vi "Agilent Oscilloscope data download.vi"() -> ()   [LabVIEW 2011]
uses:
  <vilib>/Instr/_visa.llb/VISA Open Access Mode.ctl
  <vilib>/Instr/_visa.llb/VISA Set IO Buffer Mask.ctl
panel:
  in  "run time (ms)":u32=1000
  out "error out":errorcluster
  in  "VISA GPIB Resource":refnum<visa-resource-name>="GPIB0::7::INSTR"
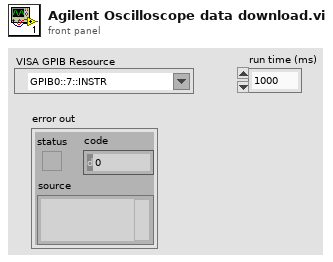
[diagram p1: front panel]
types:
  T1 = typedef "VISA Set IO Buffer Mask.ctl" = u16
  T2 = typedef "VISA Open Access Mode.ctl" = u32
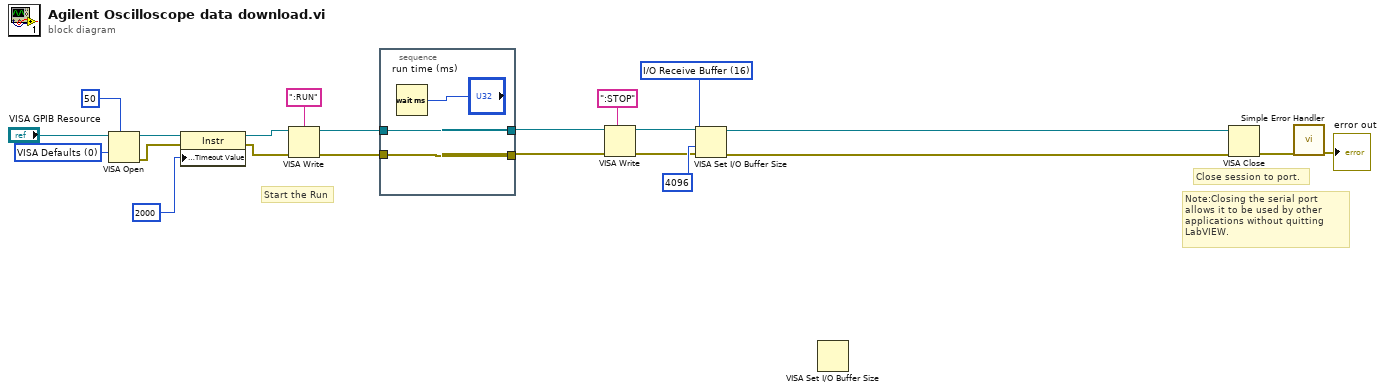
[diagram p0: block diagram]
diagram:
  w5 = T1 16 items=["I/O Receive Buffer"=16, "I/O Transmit Buffer"=32, "I/O Receive and Transmit Buffer"=48] ("Mask")
  w15 = T2 0 items=["VISA Defaults"=0, "Exclusive Lock"=1, "Load Configured Settings"=4] ("Access Mode")
  # "Start the Run"
  # "Note:Closing the serial port allows it to be used by other applications without quitting LabVIEW."
  # "Close session to port."
  n1 = VISA Open(timeout (0)=u32 50 ("VISA Open timeout (0)"), access mode=w15, VISA resource name="VISA GPIB Resource") -> (VISA resource name=w18:refnum<visa-resource-name>, error out=w17:errorcluster)  [unwired: 2 in]
  n2 = property class="Instr"(reference=w18, error in=w17, "General Settings:Timeout Value"=u32 2000) -> (reference out=w14:refnum<visa-resource-name>, error out=w13:errorcluster)
  n3 = VISA Write(VISA resource name=w14, write buffer=":RUN" ("string to write"), error in (no error)=w13) -> (VISA resource name out=w10:refnum<visa-resource-name>, error out=w8:errorcluster)  [unwired: 1 out]
  n4 = stacked-sequence {
    tunnel: w10 -> [w24]
    tunnel: [w24] -> w9
    tunnel: w8 -> [w23]
    tunnel: [w23] -> w7
    frame #0 {
      n5 = Wait (ms)(milliseconds to wait="run time (ms)") -> ()  [unwired: 1 out]
    }
  }
  n6 = VISA Write(VISA resource name=w9, write buffer=":STOP" ("string to write"), error in (no error)=w7) -> (VISA resource name out=w6:refnum<visa-resource-name>, error out=w3:errorcluster)  [unwired: 1 out]
  n7 = VISA Set I/O Buffer Size(VISA resource name=w6, mask (16)=w5, size (4096)=u32 4096, error in (no error)=w3) -> (VISA resource name out=w2:refnum<visa-resource-name>, error out=w1:errorcluster)
  n8 = VISA Set I/O Buffer Size() -> ()  [unwired: 4 in, 2 out]
  n9 = VISA Close(VISA resource name=w2, error in (no error)=w1) -> (error out=w22:errorcluster)
  n10 = call <vilib>:"Simple Error Handler.vi"("error in (no error)"=w22) -> ("error out"=→"error out":errorcluster)  [unwired: 1 in, 7 out]
